vi "XML writeSamplesToXml.vi"(11 "Sample":T1[](array[typedef])) -> (3 "Sample XML":string)   [LabVIEW 2011]
uses:
  Controls/PIM.API.Response.Samples.ctl
  WebEngine/LIB/MODULES/TR Module/Triasx.LIB/iQA Sweep Behavior.ctl
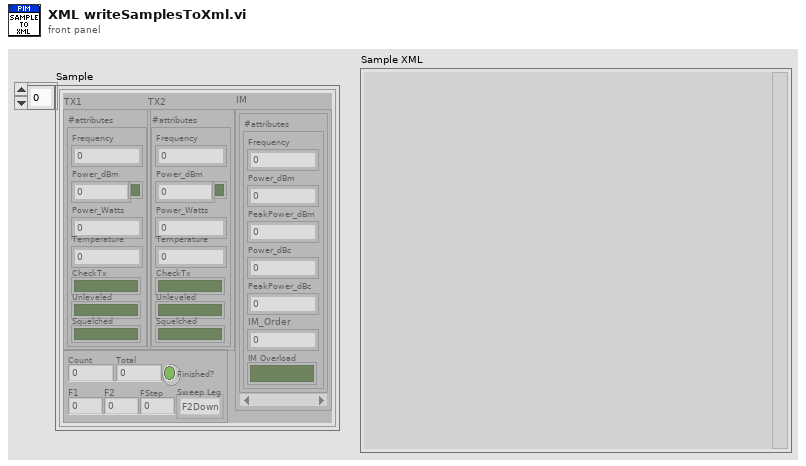
[diagram p1: front panel]
types:
  T1 = typedef "PIM.API.Response.Samples.ctl" = cluster{"TX1":cluster{"#attributes":cluster{"Frequency":dbl, "Power_dBm":dbl, "Power_Watts":dbl, "CheckTx":bool, "Unleveled":bool, "Squelched":bool, "Temperature":dbl, "ToneOn":bool}}, "TX2":cluster{"#attributes":cluster{"Frequency":dbl, "Power_dBm":dbl, "Power_Watts":dbl, "CheckTx":bool, "Unleveled":bool, "Squelched":bool, "Temperature":dbl, "ToneOn":bool}}, "IM":cluster{"#attributes":cluster{"Frequency":dbl, "Power_dBm":dbl, "PeakPower_dBm":dbl, "Power_dBc":dbl, "PeakPower_dBc":dbl, "IM_Order":u8, "IM Overload":bool}}[], "#attributes":cluster{"Count":u32, "Total":u32, "Finished?":bool, "Sweep Leg":T2, "F1":dbl, "F2":dbl, "FStep":dbl}}
  T2 = typedef "iQA Sweep Behavior.ctl" = enum16{"F2Down", "F1Up", "RxMultiIM"}
  T3 = cluster{"#attributes":cluster{"Frequency":dbl, "Power_dBm":dbl, "PeakPower_dBm":dbl, "Power_dBc":dbl, "PeakPower_dBc":dbl, "IM_Order":u8, "IM Overload":bool}}[]
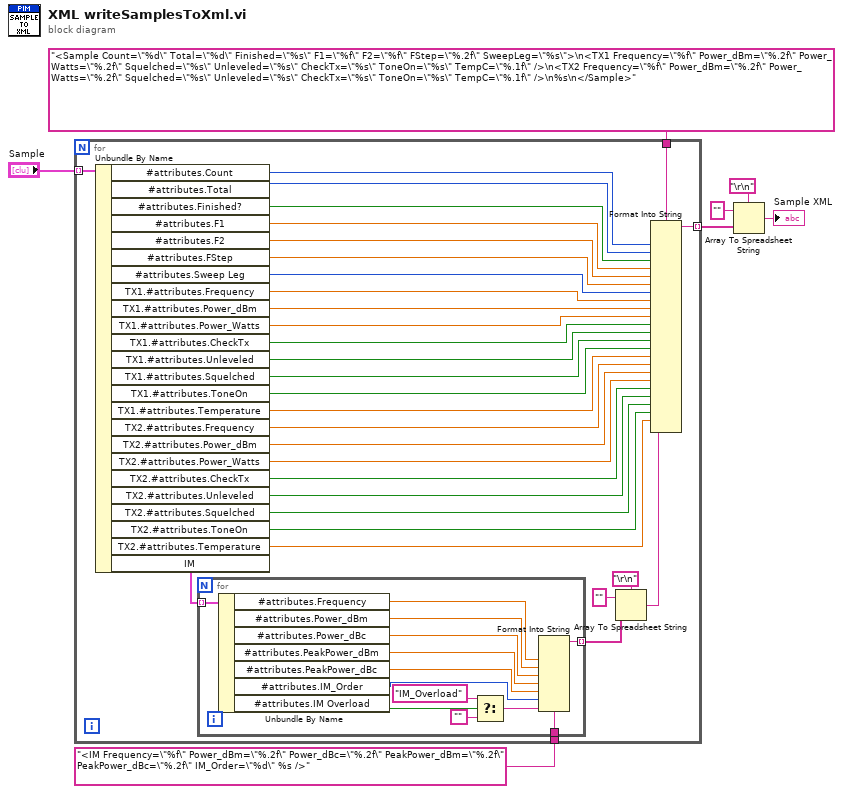
[diagram p0: block diagram]
diagram:
  n1 = for {
    tunnel: "Sample" -> [w39] mode=indexing
    tunnel: "<IM Frequency=\"%f\" Power_dBm=\"%.2f\" Power_dBc=\"%.2f\" PeakPower_dBm=\"%.2f\" PeakPower_dBc=\"%.2f\" IM_Order=\"%d\" %s />" -> [w37]
    tunnel: "<Sample Count=\"%d\" Total=\"%d\" Finished=\"%s\" F1=\"%f\" F2=\"%f\" FStep=\"%.2f\" SweepLeg=\"%s\">\n<TX1 Frequency=\"%f\" Power_dBm=\"%.2f\" Power_Watts=\"%.2f\" Squelched=\"%s\" Unleveled=\"%s\" CheckTx=\"%s\" ToneOn=\"%s\" TempC=\"%.1f\" />\n<TX2 Frequency=\"%f\" Power_dBm=\"%.2f\" Power_Watts=\"%.2f\" Squelched=\"%s\" Unleveled=\"%s\" CheckTx=\"%s\" ToneOn=\"%s\" TempC=\"%.1f\" />\n%s\n</Sample>" -> [w33]
    tunnel: [w30] -> w2 mode=indexing
    n2 = Unbundle By Name(w39) -> ("#attributes.Count"=w31:u32, "#attributes.Total"=w32:u32, "#attributes.Finished?"=w29:bool, "#attributes.F1"=w12:dbl, "#attributes.F2"=w13:dbl, "#attributes.FStep"=w14:dbl, "#attributes.Sweep Leg"=w15:T2, "TX1.#attributes.Frequency"=w16:dbl, "TX1.#attributes.Power_dBm"=w17:dbl, "TX1.#attributes.Power_Watts"=w18:dbl, "TX1.#attributes.CheckTx"=w19:bool, "TX1.#attributes.Unleveled"=w20:bool, "TX1.#attributes.Squelched"=w21:bool, "TX1.#attributes.ToneOn"=w9:bool, "TX1.#attributes.Temperature"=w11:dbl, "TX2.#attributes.Frequency"=w22:dbl, "TX2.#attributes.Power_dBm"=w23:dbl, "TX2.#attributes.Power_Watts"=w24:dbl, "TX2.#attributes.CheckTx"=w25:bool, "TX2.#attributes.Unleveled"=w26:bool, "TX2.#attributes.Squelched"=w27:bool, "TX2.#attributes.ToneOn"=w8:bool, "TX2.#attributes.Temperature"=w10:dbl, "IM"=w38:T3)
    n3 = for {
      tunnel: w38 -> [w52] mode=indexing
      tunnel: w37 -> [w48]
      tunnel: [w40] -> w34 mode=indexing
      n4 = Unbundle By Name(w52) -> ("#attributes.Frequency"=w41:dbl, "#attributes.Power_dBm"=w42:dbl, "#attributes.Power_dBc"=w43:dbl, "#attributes.PeakPower_dBm"=w44:dbl, "#attributes.PeakPower_dBc"=w45:dbl, "#attributes.IM_Order"=w46:u8, "#attributes.IM Overload"=w49:bool)
      n5 = Select(t="IM_Overload", s=w49, f="") -> (s? t:f=w47:string)
      n6 = Format Into String(format string=w48, w41, w42, w43, w44, w45, w46, w47) -> (resulting string=w40:string)  [unwired: 2 in, 1 out]
    }
    n7 = Array To Spreadsheet String(delimiter (Tab)="\r\n", array=w34, 3:"" ("format string")) -> (spreadsheet string=w28:string)
    n8 = Format Into String(format string=w33, w31, w32, w29, w12, w13, w14, w15, w16, w17, w18, w19, w20, w21, w9, w11, w22, w23, w24, w25, w26, w27, w8, w10, w28) -> (resulting string=w30:string)  [unwired: 2 in, 1 out]
  }
  n9 = Array To Spreadsheet String(delimiter (Tab)="\r\n", array=w2, 3:"" ("format string")) -> (spreadsheet string=→"Sample XML":string)
